vi "MOTOR ENC.vi"() -> (1 "RIGHT MOTOR POS":fxp<+,51,11>, 2 "LEFT MOTOR POS":fxp<+,51,11>)   [LabVIEW 2019]
uses:
  <vilib>/Platform/TimedLoop/XDataNode/timing_clust.ctl
  <vilib>/Platform/TimedLoop/XDataNode/nitl_modes.ctl
  <vilib>/Platform/TimedLoop/XDataNode/wakeup.ctl
  <vilib>/rvi/Emulation/niFpgaSctlEmulationGetInTimedLoop.vi
  <vilib>/rvi/Emulation/niFpgaEmulationReportErrorSimple.vi
  <vilib>/rvi/Emulation/niFpgaGetClockAttributes.vi
  <vilib>/rvi/Emulation/niFpgaCriticalErrorInLSC.vi
  <vilib>/rvi/eio/common/nirviEmuTemplateMethod_errors.vi
  <vilib>/platform/TimedLoop/XDataNode/XDataNode.xnode
  <vilib>/eio/EIONode/EIONode.xnode
  <vilib>/Platform/TimedLoop/XDataNode/XDNodeRunTimeDep.lvlib
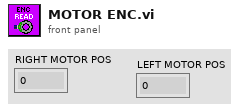
[diagram p1: front panel]
types:
  T1 = typedef "XDNodeRunTimeDep.lvlib/timing_clust.ctl" = cluster{"Expected End [f-1]":u64, "Actual End [f-1]":u64, "Finished Late? [f-1]":bool, "Expected End [i-1]":u64, "Actual End [i-1]":u64, "Finished Late? [i-1]":bool, "Expected Start [i]":u64, "Actual Start [i]":u64, "Expected Start [f]":u64, "Actual Start [f]":u64, "Source Name":string, "Structure Name":string, "Period":i64, "Deadline":i64, "Offset":i64, "Start":i64, "Priority":i32, "Timeout":i32, "Mode":T2, "Wakeup Reason":T3, "Error":errorcluster, "Source Type":string, "Secondary Source Type":string, "Global End Time":u64, "Global Start Time":u64, "Frame Duration":u64, "Iteration Duration":u64, "Assigned CPU":i32, "I/O Scan Engine Mode":u32}
  T2 = typedef "XDNodeRunTimeDep.lvlib/nitl_modes.ctl" = enum32{"No Change", "Process missed periods, maintain original phase", "Discard missed periods, maintain original phase", "Process missed periods, ignore original phase", "Discard missed periods, ignore original phase"}
  T3 = typedef "XDNodeRunTimeDep.lvlib/wakeup.ctl" = enum32{"Normal", "Aborted", "Asynchronous wakeup", "Timing source error", "Timed loop error", "Timeout"}
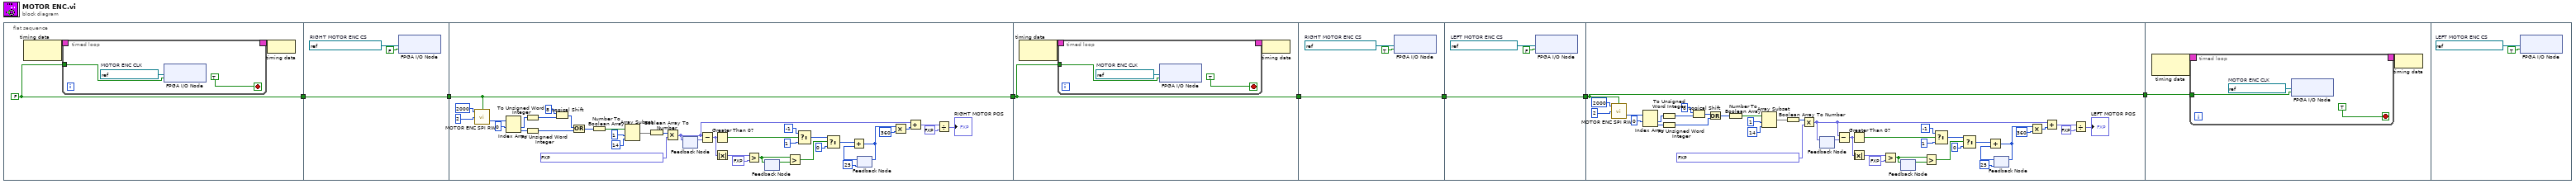
[diagram p0: block diagram]
diagram:
  n1 = flat-sequence {
    tunnel: [w8] -> w7
    tunnel: [w20] -> w6
    tunnel: w7 -> [w20]
    tunnel: w6 -> [w46]
    tunnel: [w46] -> w5
    tunnel: w5 -> [w61]
    tunnel: [w61] -> w4
    tunnel: w4 -> [w71]
    tunnel: [w71] -> w3
    tunnel: w3 -> [w76]
    tunnel: [w76] -> w2
    tunnel: w2 -> [w77]
    tunnel: [w77] -> w1
    tunnel: w1 -> [w119]
    frame #0 {
      w8 = FALSE ("CPOL")
      n2 = node-c288() -> (w10:T1)  [unwired: 1 in]
      n3 = timed-loop {
        timing: w10 -> [_]
        timing-out: [_] -> w9
        tunnel: w8 -> [w12]
        stop <- TRUE stop-if-true
        w11 = refnum<k21> "MOTOR ENC CLK"  # MOTOR ENC CLK
        n4 = xnode "FPGA I/O Node"("I/O Item"=w12, "FPGA I/O In"=w11) -> ()  [unwired: 1 out]
      }
      n5 = node-c288(w9) -> ()
    }
    frame #1 {
      w19 = refnum<k21> "RIGHT MOTOR ENC CS"  # RIGHT MOTOR ENC CS
      n6 = xnode "FPGA I/O Node"("I/O Item"=FALSE ("Value"), "FPGA I/O In"=w19) -> ()  [unwired: 1 out]
    }
    frame #2 {
      n7 = call "MOTOR ENC SPI RW.vi"("CPOL"=w46, "Frames to Write"=u8 2, "SPI Frequency (KHz)"=u16 2000 ("Frequency (kHz)")) -> ("Data Read"=w45:u8[])  [unwired: 1 in, 1 out]
      n8 = Index Array(array=w45, index #1=0 ("index")) -> (element #1=w59:u8, element #2=w58:u8)  [unwired: 1 in]
      n9 = To Unsigned Word Integer(number=w59) -> (unsigned 16bit integer=w56:u16)
      n10 = To Unsigned Word Integer(number=w58) -> (unsigned 16bit integer=w54:u16)
      n11 = Logical Shift(y=i16 8, x=w56) -> (x << y=w55:u16)
      n12 = Or(x=w55, y=w54) -> (x .or. y?=w53:u16)
      n13 = Number To Boolean Array(number=w53) -> (Boolean array=w52:bool[])
      n14 = Array Subset(array=w52, index=1, length=14) -> (w49:bool[])
      n15 = Boolean Array To Number(Boolean array=w49) -> (number=w47:u16)
      n16 = Multiply(x=w47, y=fxp<+,35,-5> 0.021973997429995507) -> (x*y=w29:fxp<+,51,11>)
      n17 = feedback #1() -> (w42:fxp<+,51,11>)  [unwired: 1 in]
      n18 = feedback-in #1(w29) -> ()
      n19 = Subtract(x=w29, y=w42) -> (x-y=w39:fxp<+/-,52,12>)
      n20 = Greater Than 0?(x=w39) -> (x > 0?=w38:bool)
      n21 = Absolute Value(x=w39) -> (abs(x)=w41:fxp<+,51,11>)
      n22 = Greater?(x=w41, y=fxp<+,51,11> 180.0) -> (0:w31:bool)
      n23 = feedback #2() -> (w32:bool)  [unwired: 1 in]
      n24 = feedback-in #2(w31) -> ()
      n25 = Greater?(x=w31, y=w32) -> (0:w30:bool)
      n26 = Select(t=i16 -1, s=w38, f=i16 1) -> (s? t:f=w37:i16)
      n27 = Select(t=w37, s=w30, f=i16 0) -> (s? t:f=w36:i16)
      n28 = feedback #3(i16 25) -> (w24:i16)
      n29 = Add(x=w36, y=w24) -> (x+y=w35:i16)
      n30 = feedback-in #3(w35) -> ()
      n31 = Multiply(x=w35, y=i16 360) -> (x*y=w34:i16)
      n32 = Add(x=w29, y=w34) -> (x+y=w33:fxp<+/-,57,17>)
      n33 = Divide(x=w33, y=fxp<+/-,57,17> 50.0) -> (x/y=→"RIGHT MOTOR POS":fxp<+/-,64,57>)
    }
    frame #3 {
      n34 = node-c288() -> (w63:T1)  [unwired: 1 in]
      n35 = timed-loop {
        timing: w63 -> [_]
        timing-out: [_] -> w62
        tunnel: w61 -> [w65]
        stop <- TRUE stop-if-true
        w64 = refnum<k21> "MOTOR ENC CLK"  # MOTOR ENC CLK
        n36 = xnode "FPGA I/O Node"("I/O Item"=w65, "FPGA I/O In"=w64) -> ()  [unwired: 1 out]
      }
      n37 = node-c288(w62) -> ()
    }
    frame #4 {
      w73 = refnum<k21> "RIGHT MOTOR ENC CS"  # RIGHT MOTOR ENC CS
      n38 = xnode "FPGA I/O Node"("I/O Item"=TRUE ("Value"), "FPGA I/O In"=w73) -> ()  [unwired: 1 out]
    }
    frame #5 {
      w75 = refnum<k21> "LEFT MOTOR ENC CS"  # LEFT MOTOR ENC CS
      n39 = xnode "FPGA I/O Node"("I/O Item"=FALSE ("Value"), "FPGA I/O In"=w75) -> ()  [unwired: 1 out]
    }
    frame #6 {
      n40 = call "MOTOR ENC SPI RW.vi"("CPOL"=w77, "Frames to Write"=u8 2, "SPI Frequency (KHz)"=u16 2000 ("Frequency (kHz)")) -> ("Data Read"=w102:u8[])  [unwired: 1 in, 1 out]
      n41 = Index Array(array=w102, index #1=0 ("index")) -> (element #1=w115:u8, element #2=w114:u8)  [unwired: 1 in]
      n42 = To Unsigned Word Integer(number=w115) -> (unsigned 16bit integer=w112:u16)
      n43 = To Unsigned Word Integer(number=w114) -> (unsigned 16bit integer=w110:u16)
      n44 = Logical Shift(y=i16 8, x=w112) -> (x << y=w111:u16)
      n45 = Or(x=w111, y=w110) -> (x .or. y?=w109:u16)
      n46 = Number To Boolean Array(number=w109) -> (Boolean array=w108:bool[])
      n47 = Array Subset(array=w108, index=1, length=14) -> (w105:bool[])
      n48 = Boolean Array To Number(Boolean array=w105) -> (number=w103:u16)
      n49 = Multiply(x=w103, y=fxp<+,35,-5> 0.021973997429995507) -> (x*y=w86:fxp<+,51,11>)
      n50 = feedback #4() -> (w99:fxp<+,51,11>)  [unwired: 1 in]
      n51 = feedback-in #4(w86) -> ()
      n52 = Subtract(x=w86, y=w99) -> (x-y=w96:fxp<+/-,52,12>)
      n53 = Greater Than 0?(x=w96) -> (x > 0?=w95:bool)
      n54 = Absolute Value(x=w96) -> (abs(x)=w98:fxp<+,51,11>)
      n55 = Greater?(x=w98, y=fxp<+,51,11> 180.0) -> (0:w88:bool)
      n56 = feedback #5() -> (w89:bool)  [unwired: 1 in]
      n57 = feedback-in #5(w88) -> ()
      n58 = Greater?(x=w88, y=w89) -> (0:w87:bool)
      n59 = Select(t=i16 -1, s=w95, f=i16 1) -> (s? t:f=w94:i16)
      n60 = Select(t=w94, s=w87, f=i16 0) -> (s? t:f=w93:i16)
      n61 = feedback #6(i16 25) -> (w81:i16)
      n62 = Add(x=w93, y=w81) -> (x+y=w92:i16)
      n63 = feedback-in #6(w92) -> ()
      n64 = Multiply(x=w92, y=i16 360) -> (x*y=w91:i16)
      n65 = Add(x=w86, y=w91) -> (x+y=w90:fxp<+/-,57,17>)
      n66 = Divide(x=w90, y=fxp<+/-,57,17> 50.0) -> (x/y=→"LEFT MOTOR POS":fxp<+/-,64,57>)
    }
    frame #7 {
      n67 = node-c288() -> (w118:T1)  [unwired: 1 in]
      n68 = timed-loop {
        timing: w118 -> [_]
        timing-out: [_] -> w117
        tunnel: w119 -> [w121]
        stop <- TRUE stop-if-true
        w120 = refnum<k21> "MOTOR ENC CLK"  # MOTOR ENC CLK
        n69 = xnode "FPGA I/O Node"("I/O Item"=w121, "FPGA I/O In"=w120) -> ()  [unwired: 1 out]
      }
      n70 = node-c288(w117) -> ()
    }
    frame #8 {
      w128 = refnum<k21> "LEFT MOTOR ENC CS"  # LEFT MOTOR ENC CS
      n71 = xnode "FPGA I/O Node"("I/O Item"=TRUE ("Value"), "FPGA I/O In"=w128) -> ()  [unwired: 1 out]
    }
  }
